vi "AuthenticateUser.vi"(3 "Password":string, 4 "Username":string, 5 "Path":path) -> (1 "Authenticated?":bool)   [LabVIEW 2025]
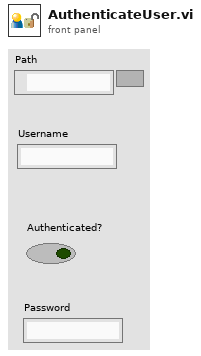
[diagram p1: front panel]
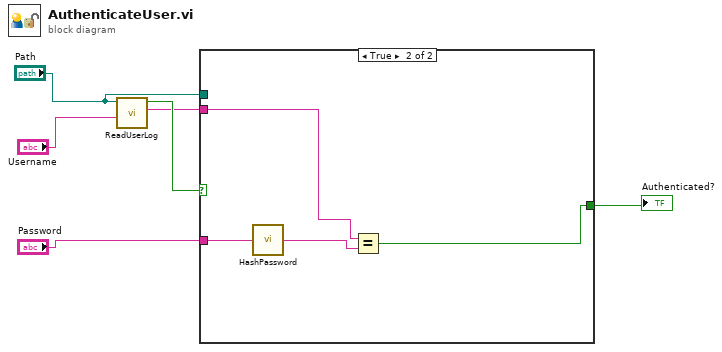
[diagram p0: block diagram]
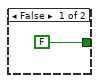
[diagram p2: hidden frame]
diagram:
  n1 = call "ReadUserLog.vi"("Username"="Username", "file path (use dialog)"="Path") -> ("Hashed Password"=w1:string, "Found?"=w5:bool)  [unwired: 2 in, 2 out]
  n2 = case shown="True" w5 {
    tunnel: [FALSE w8] -> w4
    tunnel: "Password" -> [_ w11]
    tunnel: "Path" -> [_ _]
    tunnel: w1 -> [_ w9]
    frame False {
    }
    frame True {
      n3 = call "HashPassword.vi"("Password"=w11) -> ("Hashed Password"=w10:string)
      n4 = Equal?(x=w9, y=w10) -> (x = y?=w8:bool)
    }
  }
  "Authenticated?" <- w4
